vi "Initialization Globals.vi"() -> ()   [LabVIEW 2019]
uses:
  Enum_FileNewInterval.ctl
panel:
  in  "9224 Offset":dbl[](array[numeric])=[0.005434, 0.0939, 0.1442, -0.01812, 0.0807, 0.0585, 0.0, 0.0]
  in  "9224 Scale":dbl[](array[numeric])=[0.083247, 0.08321, 0.083389, 0.083762, 0.082997, 0.083616, 1.0, 1.0]
  in  "9237 Offset":dbl[](array[numeric])=[-56.553819222701264, -42.37133513503923, 1.28, 0.0]
  in  "9237 Scale":dbl[](array[numeric])=[248170.0166994616, 256019.888229079, 10692.8714, 1.0] format="%#_6e"
  out "Nm/V Scale":dbl=17.57
  out "Damping Coef. (Nm-s/rad)":dbl=-60.0
  out "Encoder ppr":dbl=8192.0
  in  "MQTT Published Topic 2":string="/na"
  in  "MQTT Published Topic 1":string="sense"
  in  "MQTT Subscribed Topic 1":string="send"
  in  "MQTT Broker Address":string="10.10.0.129"
  out "Watchdog Enable":bool
  in  "Stbd 3 Phase Current Scaling":dbl[](array[numeric])=[2.5, 2.5, 2.5]
  in  "Stbd 3 Phase Voltage Scaling":dbl[](array[numeric])=[100.0, 100.0, 100.0]
  out "AWS Enable Upload (TDMS)":bool
  in  "Scaling Factors Grp0":dbl[](array[numeric])
  in  "PowGrp0 samples per channel":i32=500
  in  "PowGrp0 sample rate [Hz]":dbl=50000.0 format="%0.2f"
  out "Save Raw Data (3ph only)":bool=TRUE
  out "Raw Interval Time Remaining":dbl format="%<%H:%M:%S%1u>t"
  out "Raw Sampling Time Remaining":dbl format="%<%H:%M:%S%1u>t"
  out "Save Raw Data":bool=TRUE
  out "Raw Data Mode":string="Continuous"
  out "Raw Sampling Time (min)":i32=1
  out "Raw Interval (min)":i32=10
  in  "Data Folder Path":string="/media/sdb1/data"
  in  "Config File Path":string="/media/sdb1"
  out "AWS Enable Upload (Summary)":bool
  in  "AWS Bucket":string="AWS Bucket"
  in  "AWS Secret Key":string="AWS Secret Key"
  in  "AWS Access Key":string="AWS Access Key"
  out "Summary Upload Interval pow (min)":i32=10
  in  "Local file path (pow)":string="/media/sdb1/data/UPLOAD/"
  in  "Destination write path (pow)":string="/PowNow.txt"
  in  "File Write Interval":T1
  out "CSV Loop Delay (ms)":i32=500
  out "CSV Avg Time (Sec)":i32=600
  out "Enable CSV Summary File?":bool=TRUE
  out "Summary Upload Interval pos (min)":i32=10
  out "FTP Delete After Upload?":bool
  out "Enable FTP?":bool
  in  "Destination write path (pos)":string="/now.txt"
  in  "Local file path (pos)":string="/media/sdb1/data/UPLOAD/"
  in  "FTP Password":string="fakepassword"
  in  "FTP User":string="modaq1@your_Server.com"
  in  "FTP Host":string="modaq.your_Server.com"
  out "Send Alert Email":bool
  out "Email Password":string="SMTP Password"
  out "Email Username":string="modaq@your_email.com"
  out "Outgoing SMTP":string="smtp.your_email.com"
  out "Sender Email":string="MODAQ@your_email.com"
  out "Email DL 1":string="robert.raye@nrel.gov"
  out "Email DL 2":string="robert.raye@nrel.gov,\nuser1@your_email.com"
  out "Enable Email Alerts?":bool
  out "AWOL Snooze":dbl=15.0
  out "Red Snooze":dbl=60.0
  out "Yellow Snooze":dbl=60.0
  out "AWOL Radius":dbl=5.0
  out "Red Radius":dbl=2.5
  out "Yellow Radius":dbl=2.0
  out "Set Point Lon":dbl=-105.228346
  out "Set Point Lat":dbl=39.9132
  out "Watchdog Period":u32=2000
  out "Reset target on WD TO":bool
  # "I/O Configs"
  # "Watch Circle"
  # "Files and Uploads"
  # "PT-EN0-1001"
  # "PT-EN0-1002"
  # "PT-EN0-1003"
  # "CT-EN0-1001"
  # "CT-EN0-1002"
  # "CT-EN0-1003"
  # "ADD to Configurator"
  # "Watchdog Timer"
  # "Control Setpoints and Thresholds"
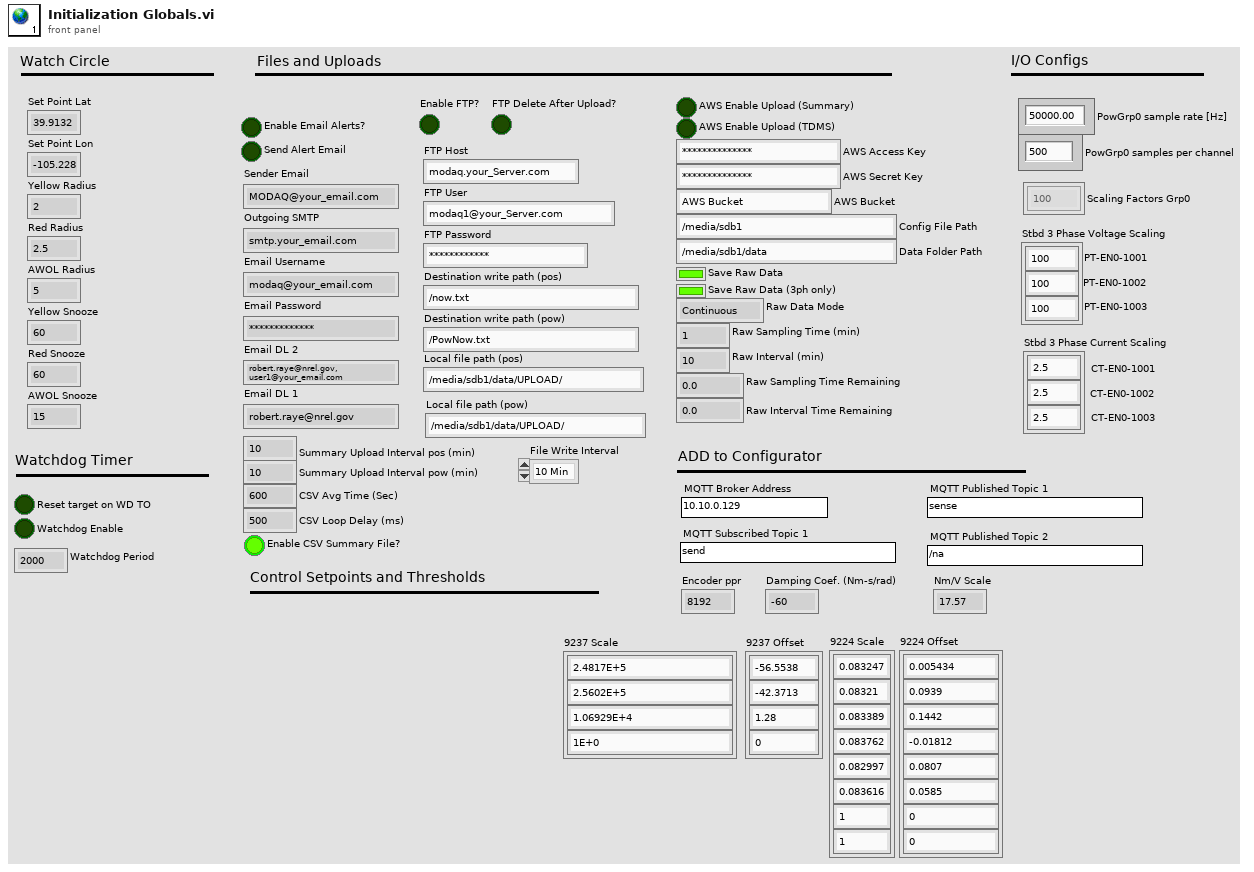
[diagram p1: front panel]
types:
  T1 = typedef "Enum_FileNewInterval.ctl" = enum16{"10 Min", "Hourly", "Daily", "Weekly", "Monthly"}
diagram:
